vi "Distance Per Counts Conversion.vi"(10 "Counts Per Rev":dbl, 11 "WheelDiameter":dbl) -> (3 "Distance/Count":dbl)   [LabVIEW 2013]
doc: "Multiplies wheel diameter by pi then divides by Counts/Revs. Returns Distance/Count"
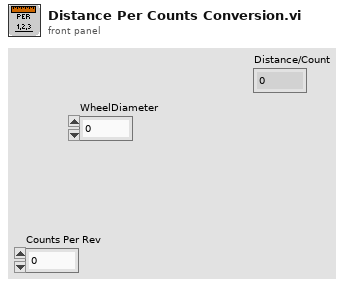
[diagram p1: front panel]
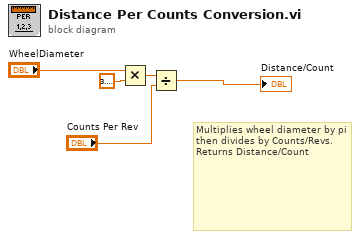
[diagram p0: block diagram]
diagram:
  # "Multiplies wheel diameter by pi then divides by Counts/Revs.  Returns Distance/Count"
  n1 = Multiply(x="WheelDiameter", y=3.141592653589793) -> (x*y=w3:dbl)
  n2 = Divide(x=w3, y="Counts Per Rev") -> (x/y=→"Distance/Count":dbl)
